vi "READ Data.vi"(8 "error in (no error)":errorcluster caption="错误输入（无错误）", 11 "THM-V6数字型温湿度 输入":refnum<class "THM-V6数字型温湿度.lvclass">) -> (0 "error out":errorcluster caption="错误输出", 3 "THM-V6数字型温湿度 输出":refnum<class "THM-V6数字型温湿度.lvclass">)   [LabVIEW 2016, in "THM-V6数字型温湿度.lvlib" / "THM-V6数字型温湿度.lvclass"]
uses:
  <vilib>/Plasmionique/MB Master/MB Master.lvlib
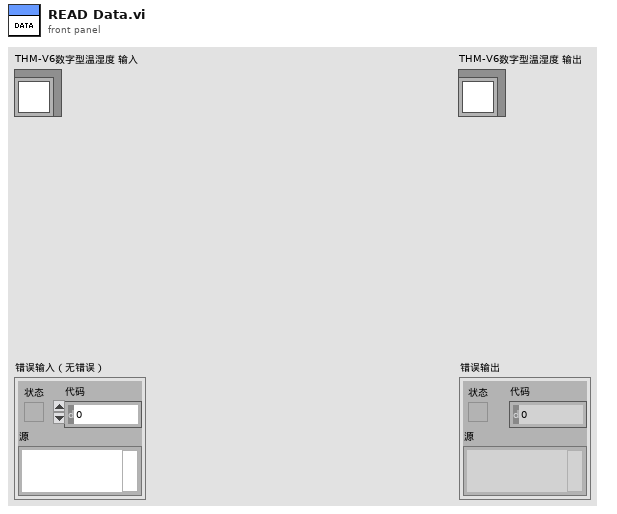
[diagram p1: front panel]
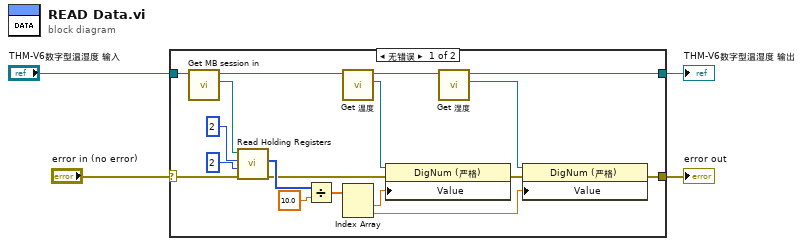
[diagram p0: block diagram]
diagram:
  n1 = case shown="无错误" "error in (no error)" {
    selector: "error in (no error)" -> [w6 w24]
    tunnel: [w5 w24] -> w3
    tunnel: [w15 w23] -> w1
    tunnel: "THM-V6数字型温湿度 输入" -> [w22 w23]
    frame No Error {
      n2 = call "Get MB session in.vi"("THM-V6数字型温湿度 in"=w22) -> ("MB Serial Master:MB_Master"=w21:refnum<class "MB_Master.lvclass">, "THM-V6数字型温湿度 out"=w20:refnum<class "THM-V6数字型温湿度.lvclass">)  [unwired: 9 in]
      n3 = call <vilib>:"Read Holding Registers.vi"("error in (no error)"=w6, "quantity"=u16 2, "starting address"=u16 2, "MB session in"=w21) -> ("error out"=w7:errorcluster, "Registers"=w12:u16[])  [unwired: 5 in, 1 out]
      n4 = Divide(x=w12, y=10.0) -> (x/y=w10:dbl[])
      n5 = call "Get 温度.vi"("THM-V6数字型温湿度 in"=w20) -> ("温度"=w18:refnum<vi>, "THM-V6数字型温湿度 out"=w19:refnum<class "THM-V6数字型温湿度.lvclass">)  [unwired: 9 in]
      n6 = Index Array(array=w10) -> (element #1=w9:dbl, element #2=w8:dbl)  [unwired: 2 in]
      n7 = property class="DigNum (严格)"(reference=w18, error in=w7, "Value"=w9) -> (error out=w16:errorcluster)  [unwired: 1 out]
      n8 = call "Get 湿度.vi"("THM-V6数字型温湿度 in"=w19) -> ("湿度"=w17:refnum<vi>, "THM-V6数字型温湿度 out"=w15:refnum<class "THM-V6数字型温湿度.lvclass">)  [unwired: 9 in]
      n9 = property class="DigNum (严格)"(reference=w17, error in=w16, "Value"=w8) -> (error out=w5:errorcluster)  [unwired: 1 out]
    }
    frame Error {
    }
  }
  "error out" <- w3
  "THM-V6数字型温湿度 输出" <- w1
